vi "Configure Display Color.vi"(0 "VISA resource name":refnum<visa-resource-name>, 1 "Display Type (0: Normal)":u16(ring) items=["Normal", "Invert"], 2 "Trace (1)":i32=1, 3 "Settings (0: Data Trace)":u16(ring) items=["Data Trace", "Memory Trace", "Graph Outer Frame", "Graph Grid Line", "Limit Test Result", "Limit Line", "Background"], 5 "Red (0)":i32, 7 "Green (0)":i32, 9 "Blue (0)":i32, 11 "error in (no error)":errorcluster) -> (4 "VISA resource name out":refnum<visa-resource-name>, 15 "error out":errorcluster)   [LabVIEW 2012, in "Tektronix TTR500 Series.lvlib"]
doc: "This VI sets color of specific display item."
uses:
  <instrlib>/Tektronix TTR500 Series/Tektronix TTR500 Series.lvlib
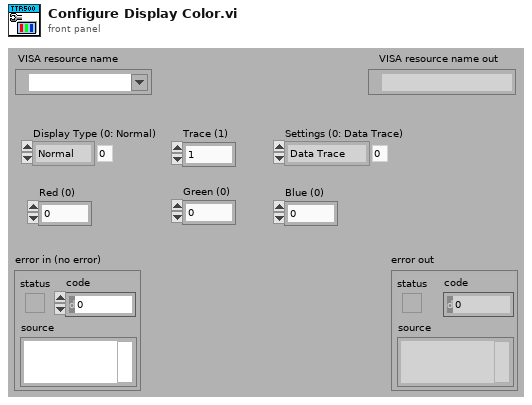
[diagram p1: front panel]
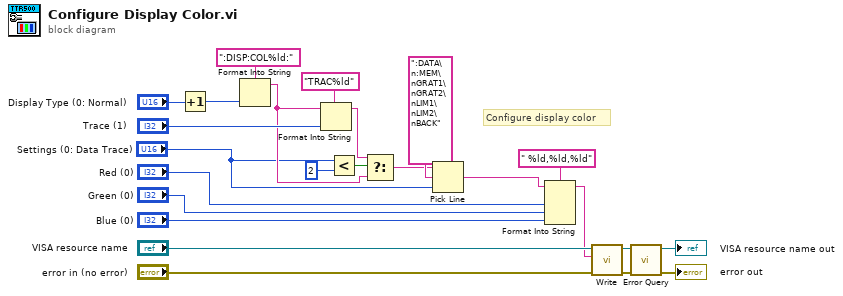
[diagram p0: block diagram]
diagram:
  # "Configure display color"
  n1 = Increment(x="Display Type (0: Normal)") -> (x+1=w5:u16)
  n2 = Format Into String(format string=":DISP:COL%ld:", w5) -> (resulting string=w9:string)  [unwired: 2 in, 1 out]
  n3 = Format Into String(format string="TRAC%ld", initial string=w9, "Trace (1)") -> (resulting string=w11:string)  [unwired: 1 in, 1 out]
  n4 = Less?(x="Settings (0: Data Trace)", y=u16 2) -> (x < y?=w12:bool)
  n5 = Select(t=w11, s=w12, f=w9) -> (s? t:f=w10:string)
  n6 = Pick Line(string ("")=w10, multi-line string=":DATA\n:MEM\nGRAT1\nGRAT2\nLIM1\nLIM2\nBACK", line index="Settings (0: Data Trace)") -> (output string=w16:string)
  n7 = Format Into String(format string=" %ld,%ld,%ld", initial string=w16, "Red (0)", "Green (0)", "Blue (0)") -> (resulting string=w8:string)  [unwired: 1 in, 1 out]
  n8 = call <instrlib>:"Write.vi"("error in (no error)"="error in (no error)", "String ()"=w8, "VISA resource name"="VISA resource name") -> ("error out"=w3:errorcluster, "VISA resource name out"=w4:refnum<visa-resource-name>)  [unwired: 6 in, 1 out]
  n9 = call <instrlib>:"Error Query.vi"("error in (no error)"=w3, "VISA resource name"=w4) -> ("error out"=→"error out":errorcluster, "VISA resource name out"=→"VISA resource name out":refnum<visa-resource-name>)  [unwired: 6 in, 2 out]
